vi "Recieve Timer Tick.vi"(8 "error in (no error)":errorcluster, 10 "Time Stamp Control":timestamp, 11 "Mag Lab Measure Controller in":refnum<class "Mag Lab Measure Controller.lvclass">) -> (0 "error out":errorcluster, 3 "Mag Lab Measure Controller out":refnum<class "Mag Lab Measure Controller.lvclass">)   [LabVIEW 2015, in "Mag Lab Measure Controller.lvclass"]
uses:
  Mag Lab Measure Controller.lvclass
  <vilib>/ActorFramework/Message Enqueuer/Message Enqueuer.lvclass
  Mag Lab Measure Controller.lvclass/Mag Lab Measure Controller.ctl
  Mag Lab Measure Base Messages/Recieve Timer Tick Msg/Recieve Timer Tick Msg.lvclass/Recieve Timer Tick Msg.ctl
  <vilib>/ActorFramework/Message Enqueuer/Message Enqueuer.lvclass/Message Enqueuer.ctl
  <vilib>/ActorFramework/Message Enqueuer/Enqueue.vi
  <vilib>/ActorFramework/Message Priority Queue/Priority Enqueue.vi
  Compound Measurement/Compound Measurement.lvclass
  Mag Lab Measure Base Messages/Recieve Timer Tick Msg/Recieve Timer Tick Msg.lvclass
panel:
  in  "Self Enqueuer":refnum<class "Message Enqueuer.lvclass">
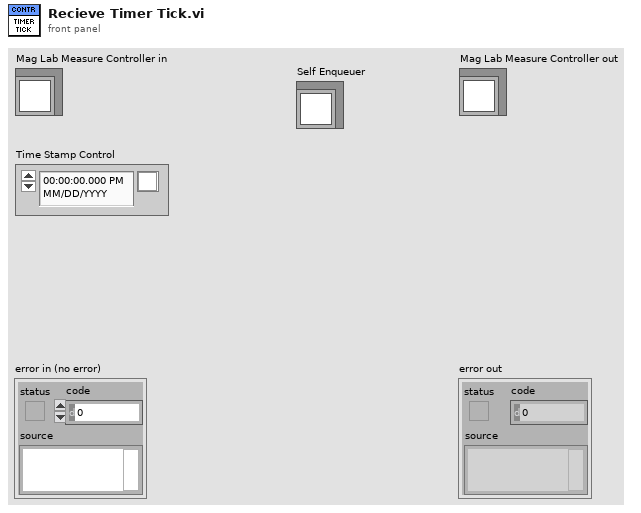
[diagram p1: front panel]
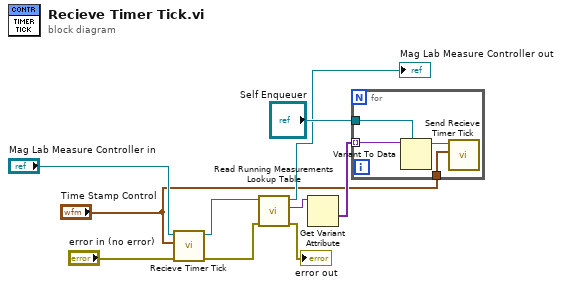
[diagram p0: block diagram]
diagram:
  n1 = call-parent "Recieve Timer Tick.vi"("error in (no error)"="error in (no error)", "Time Stamp Control"="Time Stamp Control", "Mag Lab Measurement in"="Mag Lab Measure Controller in") -> ("error out"=w5:errorcluster, "Mag Lab Measurement out"=w3:refnum<class "Mag Lab Measure Controller.lvclass">)  [unwired: 7 in]
  n2 = call "Read Running Measurements Lookup Table.vi"("error in (no error)"=w5, "Mag Lab Measure Controller in"=w3) -> ("error out"=→"error out":errorcluster, "Running Measurements Queue Lookup Table"=w8:variant, "Mag Lab Measure Controller out"=→"Mag Lab Measure Controller out":refnum<class "Mag Lab Measure Controller.lvclass">)  [unwired: 7 in]
  n3 = Get Variant Attribute(Variant=w8) -> (values=w7:variant[])  [unwired: 3 in, 3 out]
  n4 = for {
    tunnel: w7 -> [w14] mode=indexing
    tunnel: "Self Enqueuer" -> [w13]
    tunnel: "Time Stamp Control" -> [w11]
    n5 = Variant To Data(type=w13, Variant=w14) -> (data=w12:refnum<class "Message Enqueuer.lvclass">)  [unwired: 1 in, 1 out]
    n6 = call "Send Recieve Timer Tick.vi"("Time Stamp Control"=w11, "Message Enqueuer"=w12) -> ()  [unwired: 8 in, 2 out]
  }
